vi "Arrays 3.vi"() -> ()   [LabVIEW 2014]
panel:
  out "Even Numbers":i32[](array[numeric])
  in  "Max":i32
  in  "Min":i32
  # "Arrays- Third VI"
  # "Range"
  # "Even Numbers"
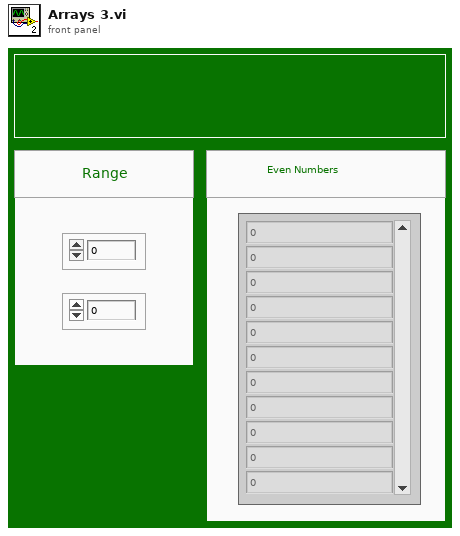
[diagram p1: front panel]
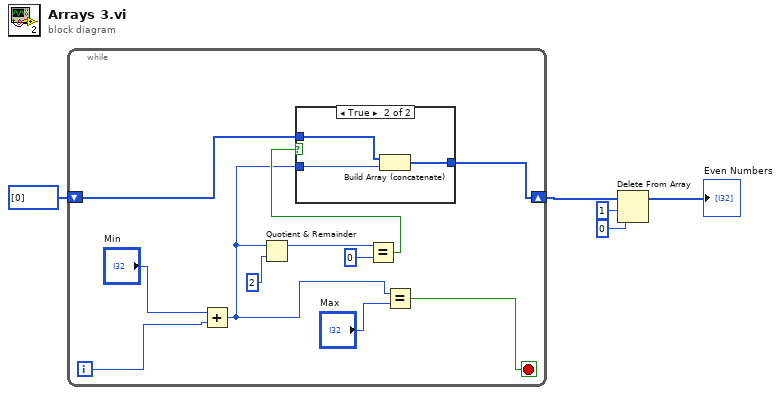
[diagram p0: block diagram]
diagram:
  n1 = while {
    shift-right: [w7] -> w5
    shift-left: i32[] [0] -> [w6]
    i -> [w15]
    stop <- w13 stop-if-true
    n2 = Add(x="Min", y=w15) -> (x+y=w8:i32)
    n3 = Quotient & Remainder(x=w8, y=2) -> (x-y*floor(x/y)=w11:i32)  [unwired: 1 out]
    n4 = Equal?(x=w11, y=0) -> (x = y?=w9:bool)
    n5 = case shown="True" w9 {
      tunnel: w8 -> [_ w20]
      tunnel: [w17 w19] -> w7
      tunnel: w6 -> [w17 w18]
      frame False {
      }
      frame True {
        n6 = Build Array (concatenate)(w18, w20) -> (w19:i32[])
      }
    }
    n7 = Equal?(x=w8, y="Max") -> (x = y?=w13:bool)
  }
  n8 = Delete From Array(array=w5, length=1, index=0) -> (array with subset deleted=→"Even Numbers":i32[])  [unwired: 1 out]
